vi "Parse Fault.vi"(1 "Buffer in":string) -> (0 "fault":string)   [LabVIEW 2019, in "PGC2D.lvlib"]
uses:
  PGC2D.lvlib
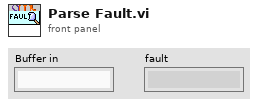
[diagram p1: front panel]
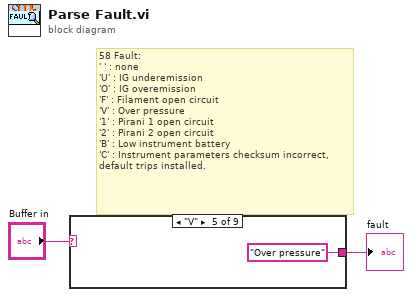
[diagram p0: block diagram]
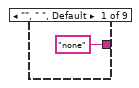
[diagram p2: hidden frame]
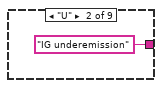
[diagram p3: hidden frame]
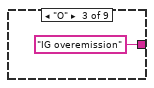
[diagram p4: hidden frame]
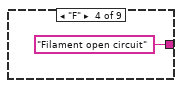
[diagram p5: hidden frame]
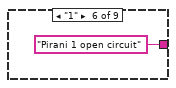
[diagram p6: hidden frame]
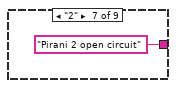
[diagram p7: hidden frame]
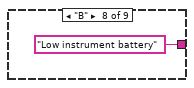
[diagram p8: hidden frame]
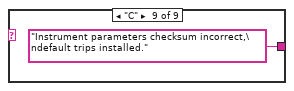
[diagram p9: hidden frame]
diagram:
  # "58 Fault:\n' ' : none\n'U' : IG underemission\n'O' : IG overemission\n'F' : Filament open circuit\n'V' : Over pressure\n'1' : Pirani 1 open circuit\n'2' : Pirani 2 open circuit\n'B' : Low instrument battery\n'C' : Instrument parameters checksum incorrect,\ndefault trips installed."
  n1 = case shown="\"V\"" "Buffer in" {
    tunnel: ["none" ("replace string (\"\")") "IG underemission" ("replace string (\"\")") "IG overemission" ("replace string (\"\")") "Filament open circuit" ("replace string (\"\")") "Over pressure" ("replace string (\"\")") "Pirani 1 open circuit" ("replace string (\"\")") "Pirani 2 open circuit" ("replace string (\"\")") "Low instrument battery" ("replace string (\"\")") "Instrument parameters checksum incorrect,\ndefault trips installed." ("replace string (\"\")")] -> w2
    frame "", " ", Default {
    }
    frame "U" {
    }
    frame "O" {
    }
    frame "F" {
    }
    frame "V" {
    }
    frame "1" {
    }
    frame "2" {
    }
    frame "B" {
    }
    frame "C" {
    }
  }
  "fault" <- w2
